vi "Configure Connection Dialog - Prototype.vi"(8 "error in (no error)":errorcluster, 9 "Current Connection":T2, 10 "Alias Mappings":T3[](array[typedef]), 11 "Possible Connections":T5(array[cluster])=[{"Resource"="", "Possible Connections"=[]}, {"Resource"="", "Possible Connections"=[]}]) -> (0 "error out":errorcluster, 1 "Connection (R,S,D)":T1, 2 "Canceled?":bool, 3 "Connection":T2)   [LabVIEW 2017, in "Routing and Faulting System Explorer.lvlib"]
uses:
  Routing and Faulting System Explorer.lvlib
  Shared/Routing and Faulting Hardware API/Types/Possible Connections for Endpoint.ctl
  Connection Row.ctl
  Shared/Alias Mapping.ctl
  Shared/Connection.ctl
  <vilib>/event_ctls.llb/lveventtype.ctl
  Shared/Routing and Faulting Hardware API/Routing and Faulting Hardware API.lvlib
  Shared/Routing and Faulting Shared.lvlib
panel:
  in  "Selected Source":string(combo)
  in  "Cancel Button":bool
  in  "OK Button":bool
  in  "Destination":string(combo)
  in  "Source":string(combo)
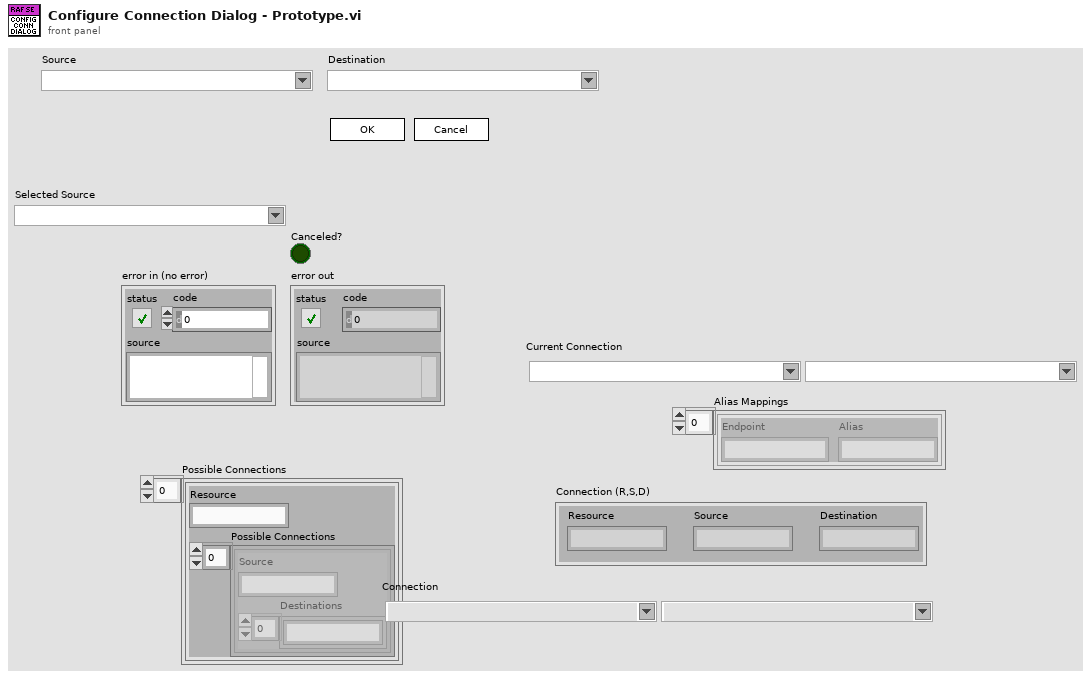
[diagram p1: front panel]
types:
  T1 = typedef "Routing and Faulting Shared.lvlib/Connection.ctl" = cluster{"Resource":string, "Source":string, "Destination":string}
  T2 = typedef "Routing and Faulting System Explorer.lvlib/Connection Row.ctl" = cluster{"Source":string, "Destination":string}
  T3 = typedef "Routing and Faulting Shared.lvlib/Alias Mapping.ctl" = cluster{"Endpoint":string, "Alias":string}
  T4 = typedef "Routing and Faulting Hardware API.lvlib/Possible Connections for Endpoint.ctl" = cluster{"Source":string, "Destinations":string[]}
  T5 = cluster{"Resource":string, "Possible Connections":T4[]}[]
  T6 = typedef "lveventtype.ctl" = enum32{"Null", "Timeout", "Annotation Menu Selection", "Annotation Menu Selection?", "App Instance Close", "App Instance Close?", "Autoscale Range Change", "Bookmark Info Change", "Cell Edit", "Cell Edit?", "Cursor Grab", "Cursor Grab?", "Cursor Menu Selection", "Cursor Menu Selection?", "Cursor Move", "Cursor Release", "Data Change", "Direction Change", "Display State Change", "Drag Ended", "Drag Enter", "Drag Leave", "Drag Over", "Drag Source Update", "Drag Starting", "Drag Starting?", "Drop", "Exec State Change", "Key Down", "Key Down?", "Key Repeat", "Key Repeat?", "Key Up", "Listbox Double Click", "Menu Activation?", "Menu Selection (App)", "Menu Selection? (App)", "Menu Selection (User)", "Mouse Down", "Mouse Down?", "Mouse Enter", "Mouse Leave", "Mouse Move", "Mouse Up", "Mouse Wheel", "NI Security User Change (App)", "Pane Size", "Panel Close", "Panel Close?", "Panel Resize", "Plot Attribute Change", "Scale Range Change", "Shortcut Menu Activation?", "Shortcut Menu Selection (App)", "Shortcut Menu Selection? (App)", "Shortcut Menu Selection (User)", "Tree Double Click", "Tree Drag", "Tree Drag?", "Tree Drop", "Tree Drop?", "Tree Item Close", "Tree Item Close?", "Tree Item Open", "Tree Item Open?", "User Event", "Value Change"}
  T7 = cluster{"Resource":string, "Possible Connections":T4[]}
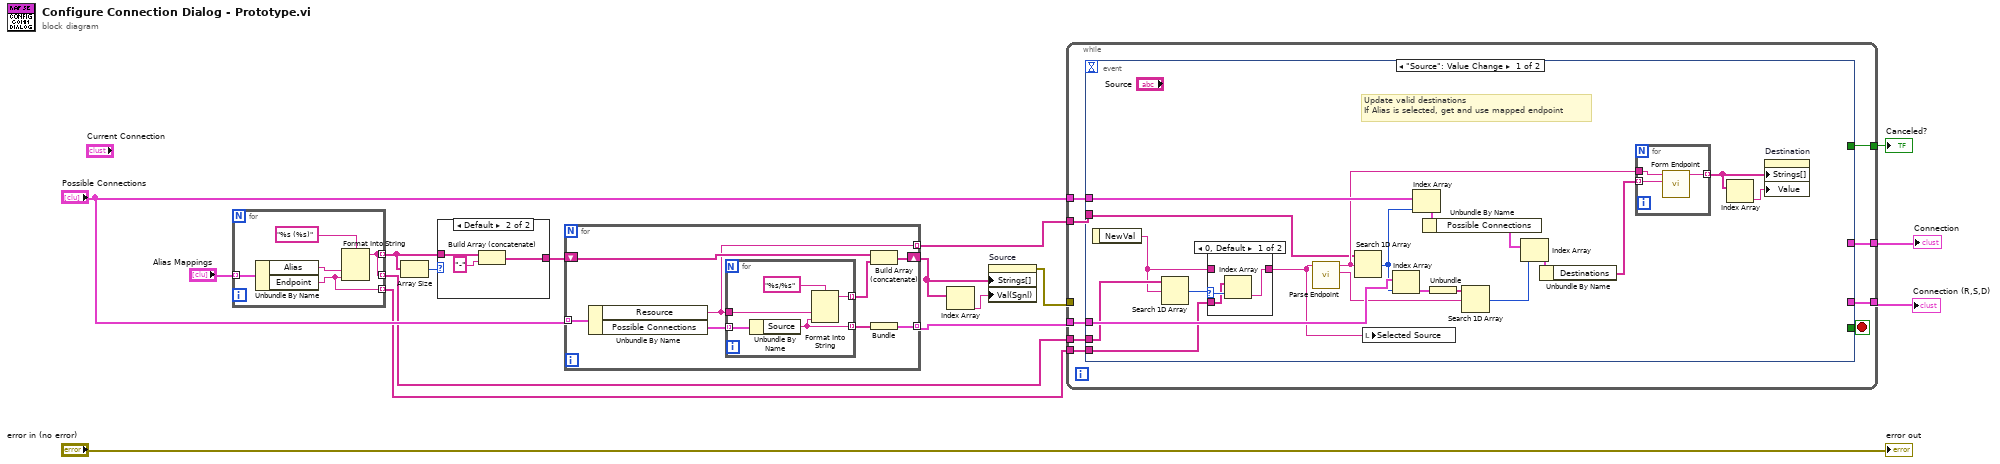
[diagram p0: block diagram]
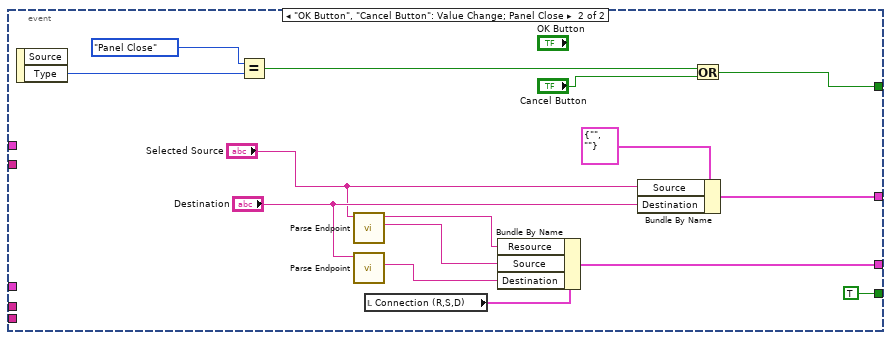
[diagram p4: hidden frame]
diagram:
  n1 = for {
    tunnel: "Alias Mappings" -> [w21] mode=indexing
    tunnel: [w17] -> w10 mode=indexing
    tunnel: [w18] -> w2 mode=indexing
    tunnel: [w17] -> w1 mode=indexing
    n2 = Unbundle By Name(w21) -> ("Alias"=w19:string, "Endpoint"=w18:string)
    n3 = Format Into String(format string="%s (%s)", w19, w18) -> (resulting string=w17:string)  [unwired: 2 in, 1 out]
  }
  n4 = Array Size(array=w10) -> (size(s)=w9:i32)
  n5 = case shown="Default" w9 {
    tunnel: w10 -> [w22 w25]
    tunnel: [w22 w23] -> w12
    frame 0 {
      # "No aliases.\nDon't add\nseparator"
    }
    frame Default {
      n6 = Build Array (concatenate)(w25, "-") -> (w23:string[])
    }
  }
  n7 = for {
    tunnel: "Possible Connections" -> [w33] mode=indexing
    shift-right: [w30] -> w5
    shift-left: w12 -> [w32]
    tunnel: [w29] -> w11 mode=indexing
    tunnel: [w26] -> w8 mode=indexing
    n8 = Unbundle By Name(w33) -> ("Resource"=w29:string, "Possible Connections"=w28:T4[])
    n9 = for {
      tunnel: w29 -> [w37]
      tunnel: [w36] -> w31 mode=indexing
      tunnel: w28 -> [w35] mode=indexing
      tunnel: [w34] -> w27 mode=indexing
      n10 = Unbundle By Name(w35) -> ("Source"=w34:string)
      n11 = Format Into String(format string="%s/%s", w37, w34) -> (resulting string=w36:string)  [unwired: 2 in, 1 out]
    }
    n12 = Build Array (concatenate)(w32, w31) -> (w30:string[])
    n13 = Bundle(w27) -> (w26:cluster{string[]})  [unwired: 1 in]
  }
  n14 = Index Array(array=w5) -> (element=w6:string)  [unwired: 1 in]
  n15 = property on="Source" class="CmbBox"("Strings[]"=w5, "Val(Sgnl)"=w6) -> (error out=w3:errorcluster)  [unwired: 2 in, 1 out]
  n16 = while {
    tunnel: [w46] -> w16
    tunnel: "Possible Connections" -> [w45]
    tunnel: [w44] -> w14
    tunnel: w11 -> [w43]
    tunnel: w8 -> [w42]
    tunnel: [w41] -> w4
    tunnel: w3 -> [_]
    tunnel: w2 -> [w40]
    tunnel: w1 -> [w39]
    stop <- w47 stop-if-true
    n17 = event shown="[0] \"Source\": Value Change" {
      selector: _ -> [_ _]
      dyn-events: _ -> [_ _]
      timeout: _ -> [_ _]
      tunnel: [_ TRUE] -> w47
      tunnel: [_ w82] -> w46
      tunnel: w45 -> [w67 _]
      tunnel: [_ w87] -> w44
      tunnel: w43 -> [w51 _]
      tunnel: w42 -> [w65 _]
      tunnel: [_ w80] -> w41
      tunnel: w40 -> [w49 _]
      tunnel: w39 -> [w53 _]
      event "Source": Value Change {
        # "Update valid destinations\nIf Alias is selected, get and use mapped endpoint"
        n18 = event-data() -> ("NewVal"=w50:string)  [unwired: 1 in]
        n19 = Search 1D Array(1D array=w53, element=w50) -> (index of element=w52:i32)  [unwired: 1 in]
        n20 = case shown="0, Default" w52 {
          selector: w52 -> [w70 _]
          tunnel: w50 -> [_ w71]
          tunnel: [w68 w71] -> w48
          tunnel: w49 -> [w69 _]
          frame 0, Default {
            n21 = Index Array(array=w69, index=w70) -> (element=w68:string)
          }
          frame -1 {
          }
        }
        n22 = call "Parse Endpoint.vi"("Resource/Endpoint"=w48) -> ("Endpoint"=w57:string, "Resource"=w56:string)  [unwired: 9 in]
        n23 = Search 1D Array(1D array=w51, element=w56) -> (index of element=w64:i32)  [unwired: 1 in]
        n24 = local write "Selected Source"(w48) -> ()
        n25 = Index Array(array=w65, index=w64) -> (element=w63:cluster{string[]})
        n26 = Index Array(array=w67, index=w64) -> (element=w66:T7)
        n27 = Unbundle By Name(w66) -> ("Possible Connections"=w61:T4[])
        n28 = Unbundle(w63) -> (w62:string[])
        n29 = Search 1D Array(1D array=w62, element=w57) -> (index of element=w60:i32)  [unwired: 1 in]
        n30 = Index Array(array=w61, index=w60) -> (element=w59:T4)
        n31 = Unbundle By Name(w59) -> ("Destinations"=w54:string[])
        n32 = for {
          tunnel: [w74] -> w58 mode=indexing
          tunnel: w56 -> [w73]
          tunnel: w54 -> [w72] mode=indexing
          n33 = call "Form Endpoint.vi"("Endpoint"=w72, "Resource"=w73) -> ("Resource/Endpoint"=w74:string)  [unwired: 9 in]
        }
        n34 = Index Array(array=w58) -> (element=w55:string)  [unwired: 1 in]
        n35 = property on="Destination" class="CmbBox"("Strings[]"=w58, "Value"=w55) -> ()  [unwired: 2 in, 2 out]
      }
      event "OK Button", "Cancel Button": Value Change; Panel Close {
        n36 = event-data() -> ("Type"=w85:T6)  [unwired: 1 in, 1 out]
        n37 = Equal?(x=lveventtype."Panel Close" ("Type"), y=w85) -> (x = y?=w84:bool)
        n38 = call "Parse Endpoint.vi"("Resource/Endpoint"="Selected Source") -> ("Endpoint"=w78:string, "Resource"=w79:string)  [unwired: 9 in]
        n39 = call "Parse Endpoint.vi"("Resource/Endpoint"="Destination") -> ("Endpoint"=w76:string)  [unwired: 9 in, 1 out]
        n40 = local read "Connection (R,S,D)"() -> (w81:T1)
        n41 = Bundle By Name(cluster=w81, "Resource"=w79, "Source"=w78, "Destination"=w76) -> (w80:T1)
        n42 = Bundle By Name(cluster=T2 {"Source"="", "Destination"=""} ("Connection"), "Source"="Selected Source", "Destination"="Destination") -> (w87:T2)
        n43 = Or(x=w84, y="Cancel Button") -> (x .or. y?=w82:bool)
      }
    }
  }
  "Canceled?" <- w16
  "Connection" <- w14
  "Connection (R,S,D)" <- w4
  "error out" <- "error in (no error)"
